vi "Query Audio Backends.vi"(8 "error in (no error)":errorcluster) -> (0 "error out":errorcluster, 3 "Backends":T1[](array[typedef]))   [LabVIEW 2020, in "G-Audio.lvlib"]
doc: "Queries the available audio backends. Resulting array is in priority order, where the first element is highest priority.\n\nOn Windows this will typically be WASAPI, DirectSound, and WinMM.\n\n<b>WARNING: Do not call this function from a VI running with a Preferred Execution System of 'user interface'.</b>"
uses:
  G-Audio.lvlib
  Controls/Backends.ctl
  <vilib>/Utility/error.llb/Error Cluster From Error Code.vi
  lib/g_audio_x86.dll
  lib/g_audio_x64.dll
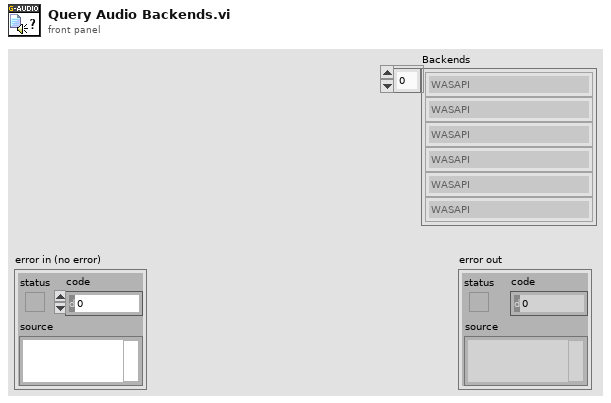
[diagram p1: front panel]
types:
  T1 = typedef "G-Audio.lvlib/Backends.ctl" = enum16{"WASAPI", "DirectSound", "WinMM", "Core Audio", "sndio", "audio(4)", "OSS", "PulseAudio", "ALSA", "JACK", "AAudio", "OpenSL|ES", "Web Audio", "Custom", "Null", "Default"}
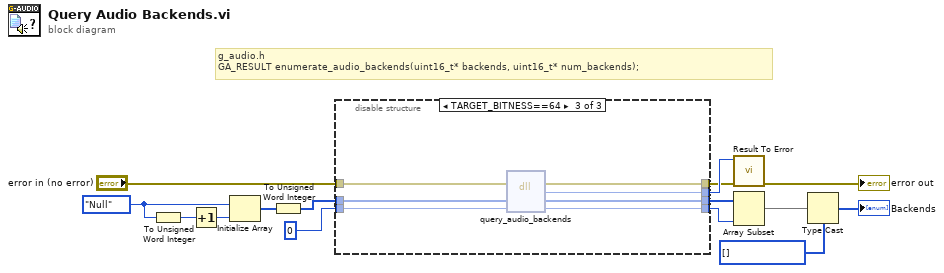
[diagram p0: block diagram]
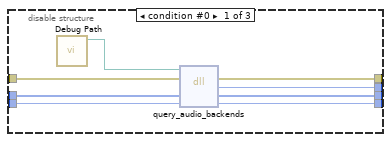
[diagram p2: hidden frame]
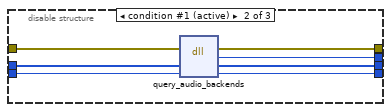
[diagram p3: hidden frame]
diagram:
  w1 = T1[] [] items=["WASAPI", "DirectSound", "WinMM", "Core Audio", "sndio", "audio(4)", "OSS", "PulseAudio", "ALSA", "JACK", "AAudio", "OpenSL|ES", "Web Audio", "Custom", "Null", "Default"]
  w11 = Backends."Null" ("Backends")
  # "g_audio.h\nGA_RESULT enumerate_audio_backends(uint16_t* backends, uint16_t* num_backends);"
  n1 = To Unsigned Word Integer(number=w11) -> (unsigned 16bit integer=w8:u16)
  n2 = Increment(x=w8) -> (x+1=w10:u16)
  n3 = Initialize Array(w11, w10) -> (w9:T1[])
  n4 = To Unsigned Word Integer(number=w9) -> (unsigned 16bit integer=w7:u16[])
  n5 = disable-structure shown="TARGET_BITNESS==64" {
    disable-tunnel: "error in (no error)" -> [w23 w30 w37]
    disable-tunnel: w7 -> [w19 w29 w35]
    disable-tunnel: [w22 w27 w36] -> w14
    disable-tunnel: u16 0 -> [w18 w28 w34]
    disable-tunnel: [w16 w24 w32] -> w4
    disable-tunnel: [w21 w26 w31] -> w15
    disable-tunnel: [w17 w25 w33] -> w5
    frame condition #0 {
      n6 = call "Debug Path.vi"() -> ("Debug Path"=w20:path)  [unwired: 11 in]
      n7 = dll-call lib="?" fn="query_audio_backends"(path in=w20, error in=w23, "backends"=w19, "num_backends"=w18) -> (error out=w22:errorcluster, "result"=w21:i32, "backends"=w17:u16[], "num_backends"=w16:u16)  [unwired: 1 in, 1 out]
    }
    frame condition #1 (active) {
      n8 = dll-call lib="C:/github/dataflowg/g-audio/src/LabVIEW/G-Audio/lib/g_audio_x86.*" fn="query_audio_backends"(error in=w30, "backends"=w29, "num_backends"=w28) -> (error out=w27:errorcluster, "result"=w26:i32, "backends"=w25:u16[], "num_backends"=w24:u16)  [unwired: 2 in, 1 out]
    }
    frame condition #2 {
      n9 = dll-call lib="C:/github/dataflowg/g-audio/src/LabVIEW/G-Audio/lib/g_audio_x64.*" fn="query_audio_backends"(error in=w37, "backends"=w35, "num_backends"=w34) -> (error out=w36:errorcluster, "result"=w31:i32, "backends"=w33:u16[], "num_backends"=w32:u16)  [unwired: 2 in, 1 out]
    }
  }
  n10 = call "Result To Error.vi"("error in (no error)"=w14, "Result Code"=w15) -> ("error out"=→"error out":errorcluster)  [unwired: 9 in]
  n11 = Array Subset(array=w5, length=w4) -> (w3:u16[])  [unwired: 1 in]
  n12 = Type Cast(type=w1, x=w3) -> (*(type *) &x=→"Backends":T1[])
